vi "se3e1.vi"() -> ()   [LabVIEW 2013]
panel:
  out "Waveform Chart":dynamicdata(graph)
  in  "Boolean":bool
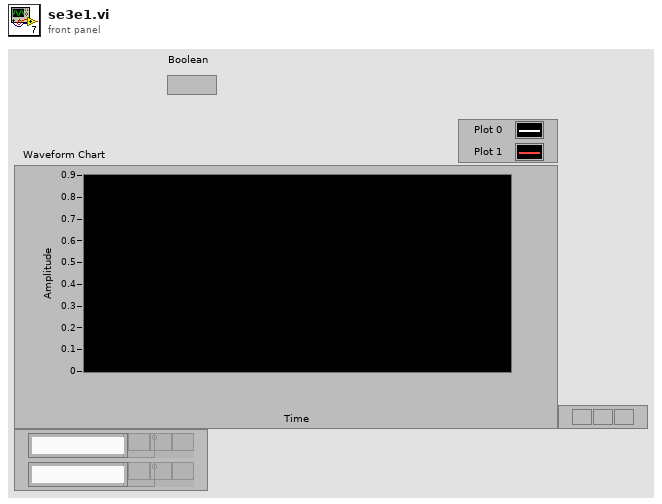
[diagram p1: front panel]
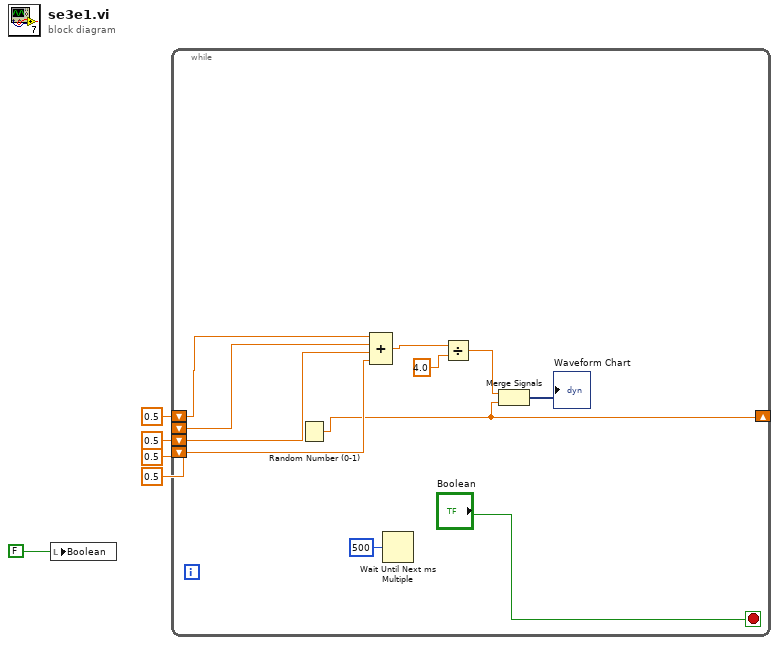
[diagram p0: block diagram]
diagram:
  n1 = local write "Boolean"(FALSE) -> ()
  n2 = while {
    shift-right: [w7] -> _
    shift-left: 0.5 ("number: 0 to 1") -> [w14]
    shift-left: 0.5 ("number: 0 to 1") -> [w15]
    shift-left: 0.5 ("number: 0 to 1") -> [w16]
    shift-left: 0.5 ("number: 0 to 1") -> [w10]
    stop <- "Boolean" stop-if-true
    n3 = Random Number (0-1)() -> (number: 0 to 1=w7:dbl)
    n4 = Compound Arithmetic op=ADD(w14, w15, w16, w10) -> (w13:dbl)
    n5 = Wait Until Next ms Multiple(millisecond multiple=u32 500) -> ()  [unwired: 1 out]
    n6 = Divide(x=w13, y=4.0) -> (x/y=w8:dbl)
    n7 = Merge Signals(w8, w7) -> (→"Waveform Chart":dynamicdata)
  }
